vi "DAQmx Scale Name.vi"(1 "DAQmx Scale Name":tag) -> (0 "DAQmx Scale Name Out":tag)   [LabVIEW 2013]
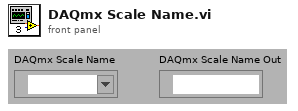
[diagram p1: front panel]
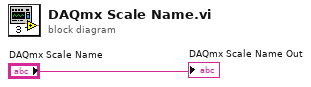
[diagram p0: block diagram]
diagram:
  "DAQmx Scale Name Out" <- "DAQmx Scale Name"
